vi "zeroHPSteps.vi"(8 "error in (no error)":errorcluster, 11 "ILCCommunications in":refnum<class "ILCCommunications.lvclass">) -> (0 "error out":errorcluster, 3 "ILCCommunications out":refnum<class "ILCCommunications.lvclass">)   [LabVIEW 2016, in "ILCCommunications.lvclass"]
uses:
  ILCCommunications.lvclass
  ILCCommunications.lvclass/ILCCommunications.ctl
  Common_RT_HPILC/HPILC/HPILC.lvclass/HPILC.ctl
  Common_RT_HPILC/HPILC/HPILC.lvclass
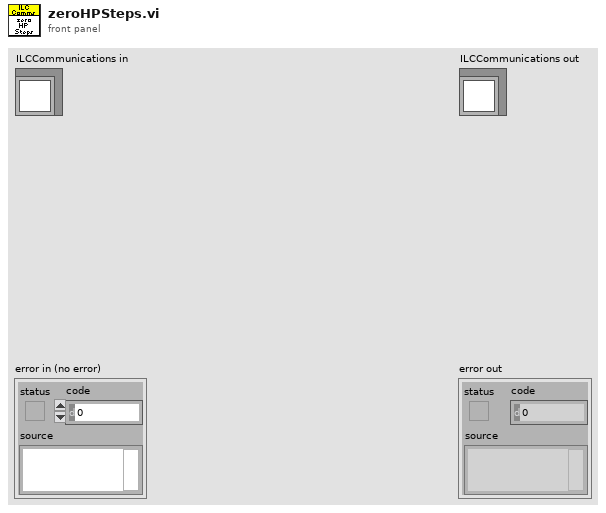
[diagram p1: front panel]
types:
  T1 = typedef "RTHPILC.lvlib/HPData.ctl" = cluster{"Constants":T2, "Command":T3, "Telemetry":T4, "Responses":T5, "Timings":T7, "Timestamps":T8}
  T2 = typedef "RTHPILC.lvlib/HPConstants.ctl" = cluster{"ID":i16, "ReferencePosition":i32, "XPosition":sgl, "YPosition":sgl, "ZPosition":sgl}
  T3 = typedef "RTHPILC.lvlib/HPCommand.ctl" = cluster{"Steps":i8}
  T4 = typedef "RTHPILC.lvlib/HPTelemetry.ctl" = cluster{"ILCFault":bool, "LimitSwitchCWOperated":bool, "LimitSwitchCCWOperated":bool, "BroadcastCounter":u8, "SSIEncoderValue":i32, "LoadCellForce":sgl}
  T5 = typedef "RTHPILC.lvlib/HPResponses.ctl" = cluster{"StepMotor":T6, "ForceAndStatus":T6}
  T6 = typedef "RTModbus.lvlib/ExceptionCodes.ctl" = u16
  T7 = typedef "RTHPILC.lvlib/HPTimings.ctl" = cluster{"BroadcastStepMotor":u32, "ForceAndStatus":u32, "FreezeSensorValues":u32, "StepMotor":u32}
  T8 = typedef "RTHPILC.lvlib/HPTimestamps.ctl" = cluster{"StepMotor":dbl, "ForceAndStatus":dbl}
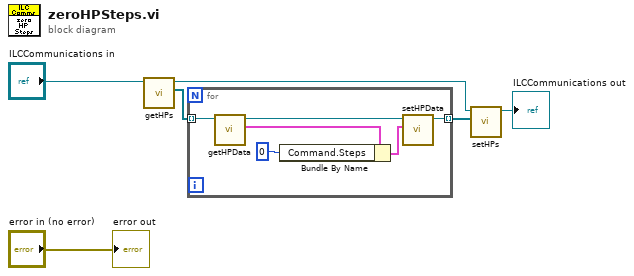
[diagram p0: block diagram]
diagram:
  n1 = call "getHPs.vi"("ILCCommunications in"="ILCCommunications in") -> ("HPs"=w6:refnum<class "HPILC.lvclass">[], "ILCCommunications out"=w4:refnum<class "ILCCommunications.lvclass">)  [unwired: 9 in]
  n2 = for {
    tunnel: w6 -> [w9] mode=indexing
    tunnel: [w7] -> w5 mode=indexing
    n3 = call "getHPData.vi"("HPILC in"=w9) -> ("HPData"=w12:T1, "HPILC out"=w8:refnum<class "HPILC.lvclass">)  [unwired: 9 in]
    n4 = Bundle By Name(cluster=w12, "Command.Steps"=i8 0) -> (w11:T1)
    n5 = call "setHPData.vi"("HPData"=w11, "HPILC in"=w8) -> ("HPILC out"=w7:refnum<class "HPILC.lvclass">)  [unwired: 9 in]
  }
  n6 = call "setHPs.vi"("HPs"=w5, "ILCCommunications in"=w4) -> ("ILCCommunications out"=→"ILCCommunications out":refnum<class "ILCCommunications.lvclass">)  [unwired: 9 in]
  "error out" <- "error in (no error)"
